vi "Update Guest Name.vi"(0 "Guest Manager UI in":refnum<class "Guest Manager UI.lvclass">, 5 "IsAvailable":bool, 7 "Guest Name":string, 11 "error in (no error)":errorcluster) -> (4 "Guest Manager UI out":refnum<class "Guest Manager UI.lvclass">, 15 "error out":errorcluster)   [LabVIEW 2023, in "Guest Manager UI.lvlib" / "Guest Manager UI.lvclass"]
uses:
  Guest Manager UI.lvclass
  Guest Manager UI.lvclass/Guest Manager UI.ctl
  Utilities/Utilities.lvlib
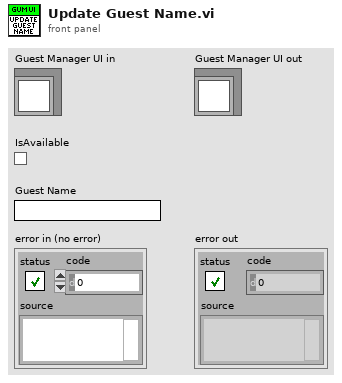
[diagram p1: front panel]
types:
  T1 = enum8{"Enabled", "Disabled", "Disabled and Grayed Out"}
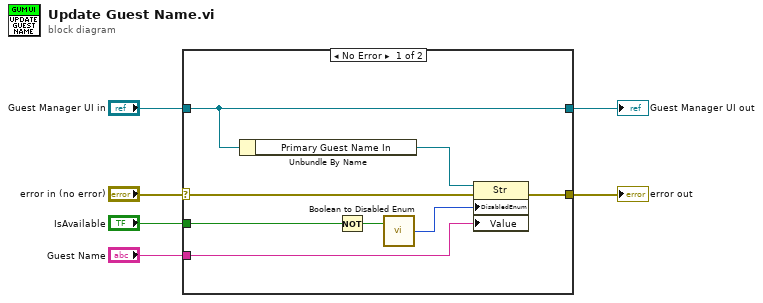
[diagram p0: block diagram]
diagram:
  n1 = case shown="No Error" "error in (no error)" {
    selector: "error in (no error)" -> [w14 w16]
    tunnel: [w13 w16] -> w5
    tunnel: [w12 w15] -> w3
    tunnel: "Guest Manager UI in" -> [w12 w15]
    tunnel: "IsAvailable" -> [w9 _]
    tunnel: "Guest Name" -> [w10 _]
    frame No Error {
      n2 = Unbundle By Name(w12) -> ("Primary Guest Name In"=w11:refnum<vi>)
      n3 = Not(x=w9) -> (.not. x?=w7:bool)
      n4 = call "Boolean to Disabled Enum.vi"("Enable"=w7) -> ("Disabled"=w8:T1)  [unwired: 1 in]
      n5 = property class="Str"(reference=w11, error in=w14, "DisabledEnum"=w8, "Value"=w10) -> (error out=w13:errorcluster)  [unwired: 1 out]
    }
    frame Error {
    }
  }
  "error out" <- w5
  "Guest Manager UI out" <- w3
